vi "takepic.vi"   [LabVIEW 2017]
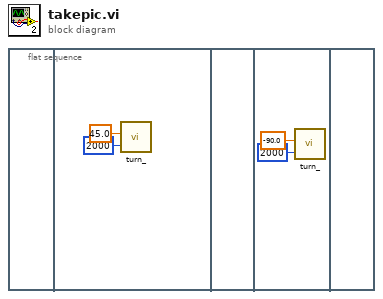
[diagram p0: block diagram]
diagram:
  n1 = flat-sequence {
    frame #0 {
    }
    frame #1 {
      n2 = call "turn_.vi"("delay"=u32 2000, "Carzeta"=45.0) -> ()  [unwired: 10 in]
    }
    frame #2 {
    }
    frame #3 {
      n3 = call "turn_.vi"("delay"=u32 2000, "Carzeta"=-90.0) -> ()  [unwired: 10 in]
    }
    frame #4 {
    }
  }
